vi "reset.vi"(8 "error in (no error)":errorcluster, 11 "DmmNiPxi in":refnum<class "DmmNi.lvclass">) -> (0 "error out":errorcluster, 3 "DmmNiPxi out":refnum<class "DmmNi.lvclass">)   [LabVIEW 2023, in "DmmNi.lvclass"]
doc: "<b>Author:</b> Wolfgang\n<b>Description:</b> This method is used to reset the instrument to a default and known state."
uses:
  DmmNi.lvclass
  DmmNi.lvclass/DmmNi.ctl
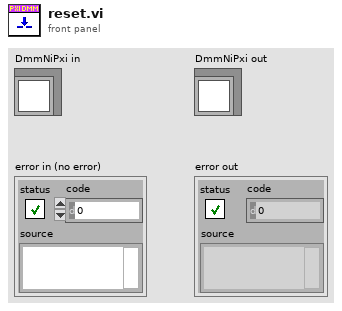
[diagram p1: front panel]
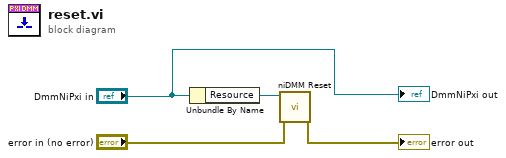
[diagram p0: block diagram]
diagram:
  n1 = Unbundle By Name("DmmNiPxi in") -> ("Resource"=w4:refnum<k15>)
  n2 = call <instrlib>:"niDMM Reset.vi"("error in (no error)"="error in (no error)", "instrument handle"=w4) -> ("error out"=→"error out":errorcluster)  [unwired: 8 in, 1 out]
  "DmmNiPxi out" <- "DmmNiPxi in"
